vi "WireCaseStructureControl.vi"(8 "error in (no error)":errorcluster, 10 "Error terminals":T1, 11 "Case structure":refnum<vi>) -> (0 "error out":errorcluster, 2 "Error terminals (dup)":T1, 3 "CaseStructure (dup)":refnum<vi>)   [LabVIEW 2017, in "ErrorStructureDrawer.lvlib"]
doc: "Moves the case structure's outer terminal to the correct vertical position for wire alignment with the error control, and draws a wire between them."
uses:
  ErrorStructureDrawer.lvlib
  Controls/ErrorTerminals.ctl
  <vilib>/Utility/miscctls.llb/LVPositionTypeDef.ctl
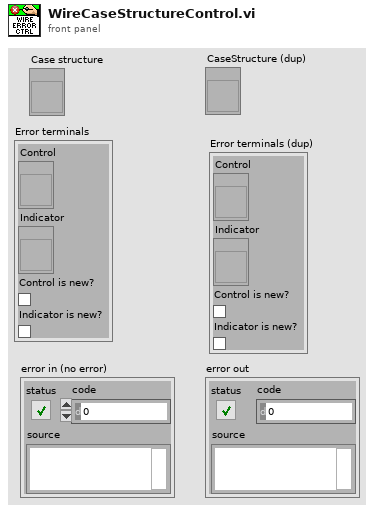
[diagram p1: front panel]
types:
  T1 = typedef "ErrorStructureDrawer.lvlib/ErrorTerminals.ctl" = cluster{"Control":refnum<vi>, "Indicator":refnum<vi>, "Control is new?":bool, "Indicator is new?":bool}
  T2 = typedef "LVPositionTypeDef.ctl" = cluster{"Left":i32, "Top":i32}
  T3 = typedef "LVRectTypeDef.ctl" = cluster{"Left":i16, "Top":i16, "Right":i16, "Bottom":i16}
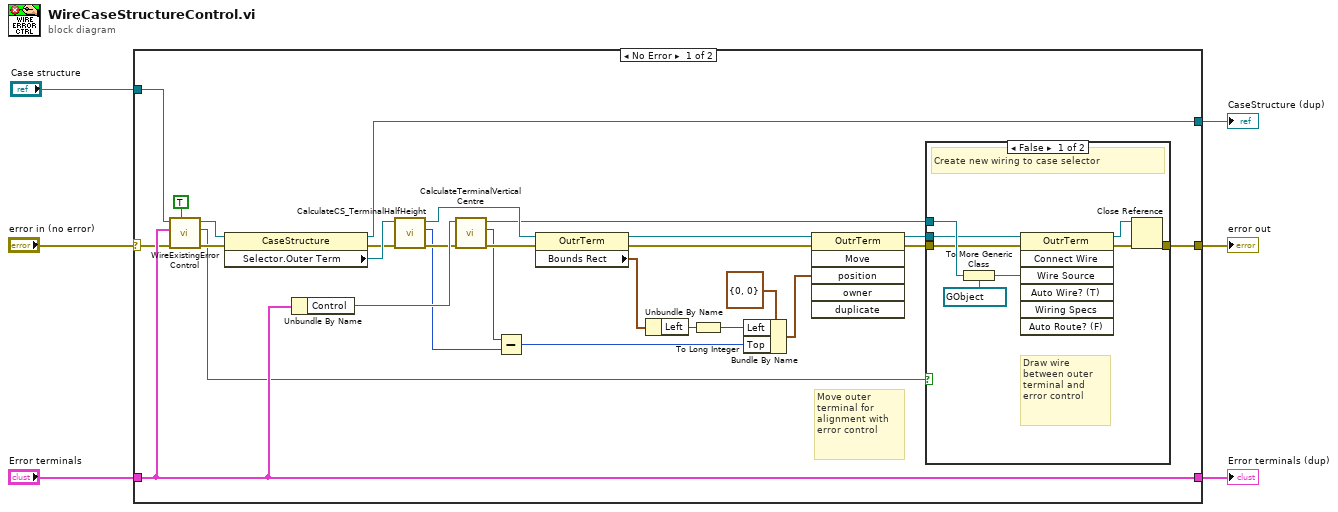
[diagram p0: block diagram]
diagram:
  n1 = case shown="No Error" "error in (no error)" {
    selector: "error in (no error)" -> [w9 w46]
    tunnel: "Error terminals" -> [w10 w44]
    tunnel: [w34 w46] -> w5
    tunnel: [w15 w45] -> w4
    tunnel: "Case structure" -> [w11 w45]
    tunnel: [w10 w44] -> w1
    frame No Error {
      # "Move outer terminal for alignment with error control"
      n2 = call "WireExistingErrorControl.vi"("Control [t] / indicator [f]"=TRUE, "error in (no error)"=w9, "Error terminals"=w10, "CaseStructure in"=w11) -> ("error out"=w13:errorcluster, "Existing wiring used?"=w8:bool, "CaseStructure (dup)"=w12:refnum<vi>)  [unwired: 4 in, 1 out]
      n3 = property class="CaseStructure"(reference=w12, error in=w13) -> (reference out=w15:refnum<vi>, error out=w21:errorcluster, "Selector.Outer Term"=w26:refnum<vi>)
      n4 = Unbundle By Name(w10) -> ("Control"=w23:refnum<vi>)
      n5 = call "CalculateCS_TerminalHalfHeight.vi"("error in (no error)"=w21, "OuterTerminal"=w26) -> ("error out"=w22:errorcluster, "CS outer terminal half-height"=w20:i32, "OuterTerminal (dup)"=w30:refnum<vi>)  [unwired: 7 in]
      n6 = call "CalculateTerminalVerticalCentre.vi"("error in (no error)"=w22, "ControlTerminal"=w23) -> ("error out"=w27:errorcluster, "Terminal's vertical centre position"=w24:i32, "ControlTerminal (dup)"=w17:refnum<vi>)  [unwired: 7 in]
      n7 = Subtract(x=w24, y=w20) -> (x-y=w33:i32)
      n8 = property class="OutrTerm"(reference=w30, error in=w27) -> (reference out=w29:refnum<vi>, error out=w28:errorcluster, "Bounds Rect"=w25:T3)
      n9 = Unbundle By Name(w25) -> ("Left"=w31:i16)
      n10 = To Long Integer(number=w31) -> (32bit integer=w32:i32)
      n11 = Bundle By Name(cluster=T2 {"Left"=0, "Top"=0} ("position"), "Left"=w32, "Top"=w33) -> (w19:T2)
      n12 = invoke class="OutrTerm" method="Move"(reference=w29, error in=w28, "position"=w19) -> (reference out=w16:refnum<vi>, error out=w14:errorcluster)  [unwired: 3 in, 4 out]
      n13 = case shown="False" w8 {
        tunnel: [w42 w43] -> w34
        tunnel: w17 -> [w37 _]
        tunnel: w16 -> [w36 _]
        tunnel: w14 -> [w35 w43]
        frame False {
          # "Draw wire between outer terminal and error control"
          # "Create new wiring to case selector"
          n14 = To More Generic Class(target class=refnum<vi> refnum ("Wire Source"), reference=w37) -> (generic class reference=w41:refnum<vi>)
          n15 = invoke class="OutrTerm" method="Connect Wire"(reference=w36, error in=w35, "Wire Source"=w41) -> (reference out=w39:refnum<vi>, error out=w38:errorcluster)  [unwired: 4 in, 5 out]
          n16 = Close Reference(reference=w39, error in (no error)=w38) -> (error out=w42:errorcluster)
        }
        frame True {
          # "Existing wiring to case selector was used, do nothing"
        }
      }
    }
    frame Error {
    }
  }
  "error out" <- w5
  "CaseStructure (dup)" <- w4
  "Error terminals (dup)" <- w1
